vi "Cycle_Calculator.vi"(7 "Cycle Specs":T1, 8 "Excitation Specs":T2) -> (0 "Samples Before Frequency Change":i32[](array[numeric]), 1 "Samples Before Measuring":i32[](array[numeric]), 2 "Samples Needed to Settle":i32[](array[numeric]), 3 "Samples for Calculation":i32[](array[numeric]), 5 "Excitation Frequencies":dbl[](array[numeric]), 6 "Total Number of Samples":i32)   [LabVIEW 2017, in "DSA.lvlib"]
doc: "Calculates a list of logmartically spaced frequencies to excite the system at, the number of samples needed to be ignored in waiting for the excitation to settle and the number of samples needed to be measured in order to calculate the frequency response for each excitation frequency.\n\nInputs: \n\n- Excitation Specs:\n - Used: Initial Frequency, Final Frequency, Frequency Units, Number of Frequencies, & Sampling Time\n - Not: Amplitude & Offset\n\n- Cycle Specs\n - Used: Cycles to Settle & Cycles to Calculate\n\nOutputs:\n\n- Excitation Frequencies: A list of logmarithically spaced frequencies to excite the system at.\n\n- Samples for Calculation: A list of the number of samples to be measured per frequency to measure the freqeuncy response.\n\n- Samples Needed to Settle: A list of the number of samples to ignore in waiting for the system to settle\n\n- Samples Before Freq. Change: A list of the indices of the last sample taken at a particular frequency before the frequency changes. The following sample, the excitaton frequency changes. \n\n- Samples Before Measuring: A list of the last sample ingored. The following sample, measuring should begin.\n\n- Total Number of Samples: The total samples (ingored + measured) needed to run the DSA."
uses:
  DSA.lvlib
  <vilib>/Analysis/NI_AALBase.lvlib
  <vilib>/Analysis/1siggen.llb/Ramp Pattern by Samples.vi
panel:
  # "Cycle_Calculator"
  # "DSA Specs"
  # "Outputs"
  # "Excitation Frequencies"
  # "Samples Needed"
  # "Measuring"
  # "Frequency Change"
  # "Per Frequency"
  # "Per Frequency"
  # "Excitation Frequencies"
  # "Frequency\nUnits"
  # "[Hz]"
  # "Excitation Magnitude"
  # "[rad/s]"
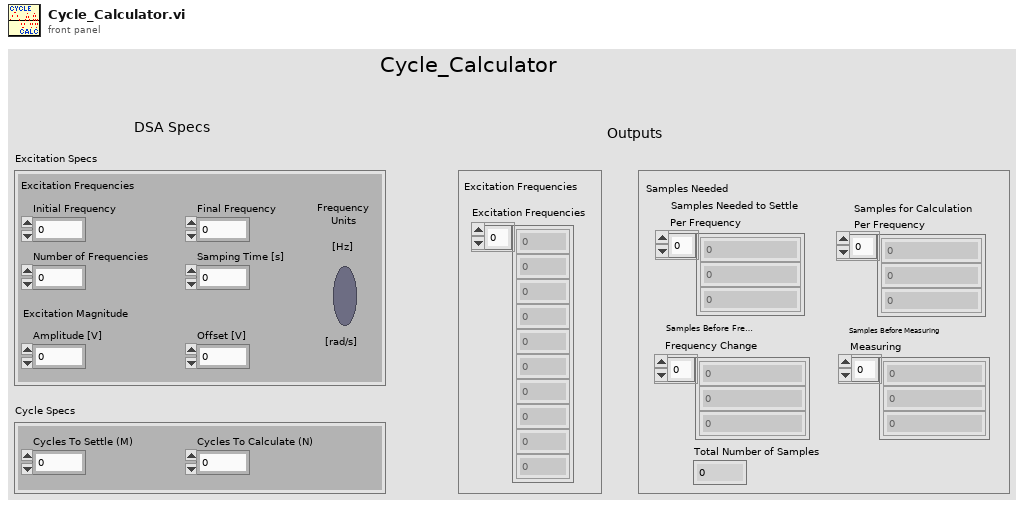
[diagram p1: front panel]
types:
  T1 = cluster{"Cycles To Settle (M)":i16, "Cycles To Calculate (N)":i16}
  T2 = cluster{"Initial Frequency":dbl, "Final Frequency":dbl, "Number of Frequencies":i16, "Samping Time [s]":dbl, "Amplitude [V]":dbl, "Offset [V]":dbl, "Freq Unit":bool}
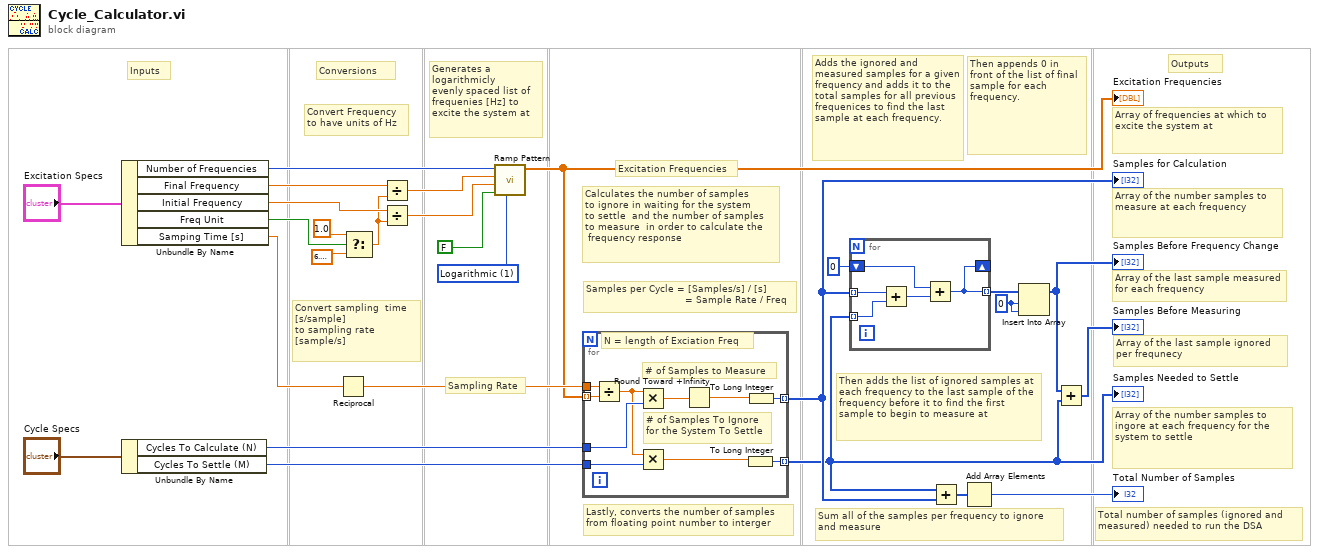
[diagram p0: block diagram]
diagram:
  w4 = 0
  w16 = u16 1 items=["Linear", "Logarithmic"] ("type")
  # "Then appends 0 in front of the list of final sample for each frequency."
  # "Then adds the list of ignored samples at each frequency to the last sample of the frequency before it to find the first sample to begin to measure at"
  # "Array of the last sample ignored per frequnecy"
  # "Adds the ignored and measured samples for a given frequency and adds it to the total samples for all previous frequenices to find the last sample at each frequency."
  # "Sum all of the samples per frequency to ignore and measure"
  # "Total number of samples (ignored and measured) needed to run the DSA"
  # "Array of the last sample measured for each frequency"
  # "Array of the number samples to ingore at each frequency for the system to settle"
  # "Array of the number samples to measure at each frequency"
  # "Array of frequencies at which to excite the system at"
  # "Lastly, converts the number of samples\nfrom floating point number to interger"
  # "Sampling Rate"
  # "Samples per Cycle = [Samples/s] / [s]\n                                 = Sample Rate / Freq"
  # "Excitation Frequencies"
  # "Outputs"
  # "Calculates the number of samples \nto ignore in waiting for the system \nto settle  and the number of samples\nto measure  in order to calculate the\n frequency response"
  # "Convert sampling  time\n[s/sample]\nto sampling rate \n[sample/s]"
  # "Conversions"
  # "Generates a\nlogarithmicly\nevenly spaced list of \nfrequenies [Hz] to\nexcite the system at"
  # "Inputs"
  # "Convert Frequency\nto have units of Hz"
  n1 = Unbundle By Name("Excitation Specs") -> ("Number of Frequencies"=w26:i16, "Final Frequency"=w25:dbl, "Initial Frequency"=w24:dbl, "Freq Unit"=w21:bool, "Samping Time [s]"=w14:dbl)
  n2 = Unbundle By Name("Cycle Specs") -> ("Cycles To Calculate (N)"=w12:i16, "Cycles To Settle (M)"=w11:i16)
  n3 = Reciprocal(x=w14) -> (1/x=w13:dbl)
  n4 = Select(t=1.0, s=w21, f=6.283185307179586) -> (s? t:f=w20:dbl)
  n5 = Divide(x=w25, y=w20) -> (x/y=w19:dbl)
  n6 = Divide(x=w24, y=w20) -> (x/y=w18:dbl)
  n7 = call-poly <vilib>:"Ramp Pattern.vi"("type"=w16, "exclude end?"=FALSE, "start"=w18, "end"=w19, "samples"=w26) -> ("Ramp Pattern"=w6:dbl[])  [unwired: 5 in, 1 out]
  "Excitation Frequencies" <- w6
  n8 = for {
    tunnel: w6 -> [w37] mode=indexing
    tunnel: w13 -> [w36]
    tunnel: w12 -> [w35]
    tunnel: w11 -> [w33]
    tunnel: [w29] -> w7 mode=indexing
    tunnel: [w28] -> w3 mode=indexing
    # "# of Samples To Ignore\nfor the System To Settle"
    # "# of Samples to Measure"
    # "N = length of Exciation Freq"
    n9 = Divide(x=w36, y=w37) -> (x/y=w34:dbl)
    n10 = Multiply(x=w34, y=w35) -> (x*y=w32:dbl)
    n11 = Multiply(x=w34, y=w33) -> (x*y=w30:dbl)
    n12 = Round Toward +Infinity(x=w32) -> (ceil(x): smallest int >= x=w31:dbl)
    n13 = To Long Integer(number=w30) -> (32bit integer=w28:i32)
    n14 = To Long Integer(number=w31) -> (32bit integer=w29:i32)
  }
  "Samples for Calculation" <- w7
  "Samples Needed to Settle" <- w3
  n15 = for {
    shift-right: [w38] -> _
    shift-left: 0 -> [w39]
    tunnel: w7 -> [w42] mode=indexing
    tunnel: w3 -> [w41] mode=indexing
    tunnel: [w38] -> w5 mode=indexing
    n16 = Add(x=w42, y=w41) -> (x+y=w40:i32)
    n17 = Add(x=w39, y=w40) -> (x+y=w38:i32)
  }
  n18 = Add(x=w3, y=w7) -> (x+y=w10:i32[])
  n19 = Add Array Elements(numeric array=w10) -> (sum=→"Total Number of Samples":i32)
  n20 = Insert Into Array(array=w5, index=w4, new element=w4) -> (w2:i32[])
  "Samples Before Frequency Change" <- w2
  n21 = Add(x=w2, y=w3) -> (x+y=→"Samples Before Measuring":i32[])
